vi "Write All Elements Hidden.vi"(8 "error in (no error)":errorcluster, 10 "Temp. params. hidden":T1={"Axis origin relative position"=0.5, "Regression file relative path"=""}, 11 "Temp params in":refnum<class "CV-Temperature.lvclass">) -> (0 "error out":errorcluster, 3 "Temp params out":refnum<class "CV-Temperature.lvclass">)   [LabVIEW 2013, in "CameraVision.lvlib" / "CV-Temperature.lvclass"]
uses:
  CV-Temperature.lvclass
  Temperature-parameters-advanced.ctl
  CV-Temperature.lvclass/CV-Temperature.ctl
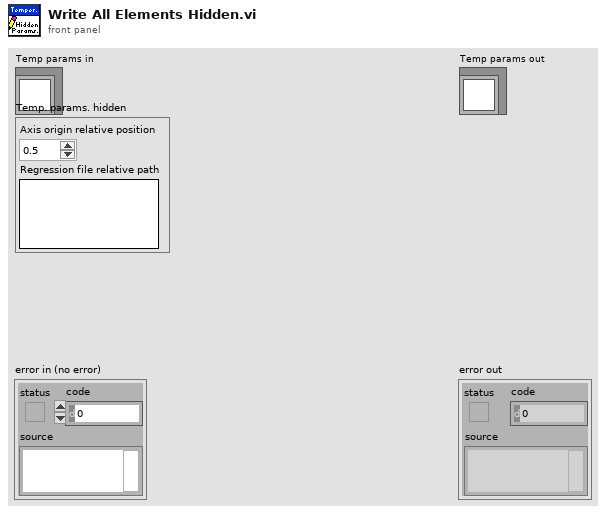
[diagram p1: front panel]
types:
  T1 = typedef "CameraVision.lvlib/CV-Temperature.lvclass/Temperature-parameters-advanced.ctl" = cluster{"Axis origin relative position":dbl, "Regression file relative path":string}
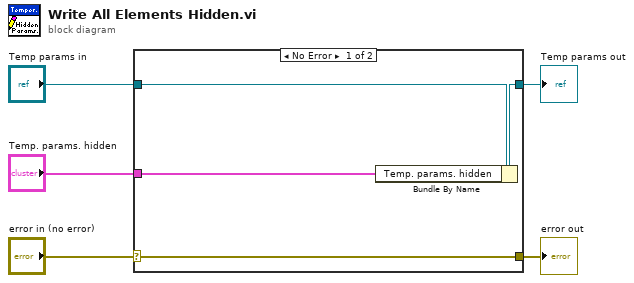
[diagram p0: block diagram]
diagram:
  n1 = case shown="No Error" "error in (no error)" {
    selector: "error in (no error)" -> [w9 w10]
    tunnel: [w9 w10] -> w4
    tunnel: [w7 w11] -> w2
    tunnel: "Temp params in" -> [w8 w11]
    tunnel: "Temp. params. hidden" -> [w6 _]
    frame No Error {
      n2 = Bundle By Name(cluster=w8, "Temp. params. hidden"=w6) -> (w7:refnum<class "CV-Temperature.lvclass">)
    }
    frame Error {
    }
  }
  "error out" <- w4
  "Temp params out" <- w2
